vi "Configure Level Trigger.vi"(6 "Enable Level Filtering (Enable)":bool=TRUE, 7 "Coupling (0:AC)":u16(ring) items=["AC", "DC"], 8 "error in (no error)":errorcluster, 9 "Percentage (0%)":dbl, 10 "Slope (1:Positive)":u16(ring)=1 items=["Negative", "Positive"], 11 "VISA resource name":refnum<visa-resource-name>) -> (0 "error out":errorcluster, 3 "VISA resource name out":refnum<visa-resource-name>)   [LabVIEW 2020, in "3458A Basic Driver.lvlib"]
doc: "Configures the DMM for what kind of level triggering will cause the instrument to start making measurements."
uses:
  3458A Basic Driver.lvlib
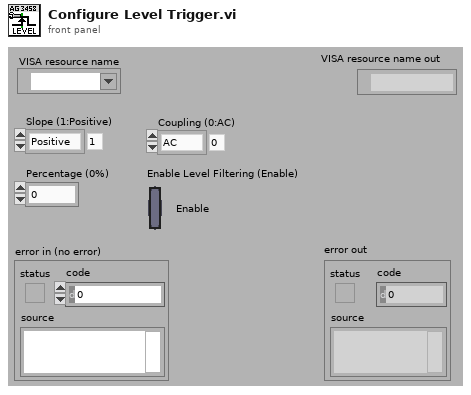
[diagram p1: front panel]
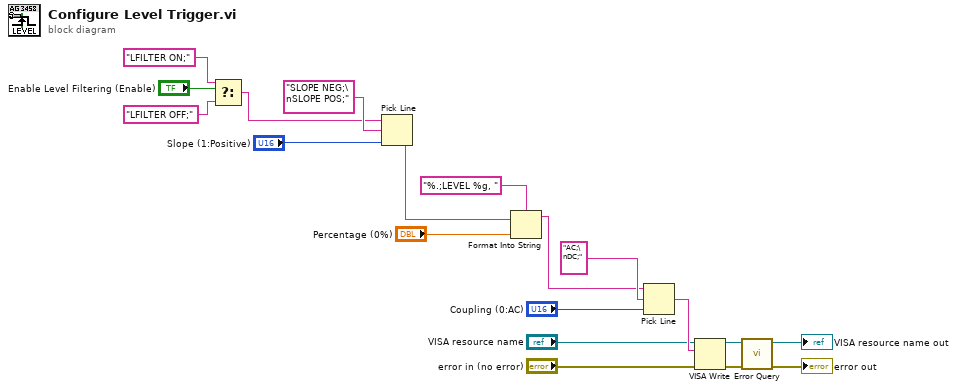
[diagram p0: block diagram]
diagram:
  n1 = Select(t="LFILTER ON;", s="Enable Level Filtering (Enable)", f="LFILTER OFF;") -> (s? t:f=w14:string)
  n2 = Pick Line(string ("")=w14, multi-line string="SLOPE NEG;\nSLOPE POS;", line index="Slope (1:Positive)") -> (output string=w13:string)
  n3 = Format Into String(format string="%.;LEVEL %g, ", initial string=w13, "Percentage (0%)") -> (resulting string=w12:string)  [unwired: 1 in, 1 out]
  n4 = Pick Line(string ("")=w12, multi-line string="AC;\nDC;", line index="Coupling (0:AC)") -> (output string=w9:string)
  n5 = VISA Write(VISA resource name="VISA resource name", write buffer=w9, error in (no error)="error in (no error)") -> (VISA resource name out=w11:refnum<visa-resource-name>, error out=w10:errorcluster)  [unwired: 1 out]
  n6 = call "Error Query.vi"("error in (no error)"=w10, "VISA resource name"=w11) -> ("error out"=→"error out":errorcluster, "VISA resource name out"=→"VISA resource name out":refnum<visa-resource-name>)  [unwired: 6 in, 2 out]
